vi "Configuration Utility.vi"() -> ()   [LabVIEW 2013, in "configuration library.lvlib"]
doc: "This is the main VI for the configuration editor."
uses:
  configuration library.lvlib
  Controls/StateCluster.ctl
  Configuration Editor/Classes/SystemConfigRepo/SystemConfigRepo.lvclass
  <vilib>/CEF_TreeControl/Node/NodeRef.ctl
  <vilib>/CEF_TreeControl/Node/NISE_CEF_Node.lvclass
  <vilib>/CEF_TreeControl/Node/UserEventRef.ctl
  <vilib>/CEF_TreeControl/Controls/EventCluster.ctl
  subVI/SplashScreen/splash screen.ctl
  subVI/SplashScreen/notifier data.ctl
  Controls/add message.ctl
  Controls/MoveMessage.ctl
  Configuration Editor/Classes/Systems/Systems.lvclass
  <vilib>/CEF_TreeControl/Repository/NISE_CEF_Repository.lvclass
  Configuration Editor/Classes/Module editor node/module editor node.lvclass
  <vilib>/NI/AMC/Create Single Message.vi
  <vilib>/NI/AMC/Update Message Routing Info.vi
  <vilib>/NI/AMC/Read Termination Message.vi
  Configuration Editor/subVIs/Glyphs Status.ctl
  Configuration Editor/subVIs/Add status to name.vi
  <vilib>/NI/AMC/Send Message.vi
  <vilib>/NI/AMC/Globals.vi
  Configuration Editor/Classes/EngineTags/EngineTags.lvclass
  Configuration Editor/Classes/Asynchronous Component Editor Node/Asynchronous Module Editor Node.lvclass
  <vilib>/NI/Module Timing Source/timing source/TBM timing source.lvclass
  Configuration Editor/Classes/TBM Configuration Node/TBM Configuration Node.lvclass
  <vilib>/NI/Tag Bus Module Framework/root configuration/TBM configuration.lvclass
  Framework Configuration Classes/target configuration/PL_Target Configuration.lvclass
  Configuration Editor/Classes/Targets/Targets.lvclass
  Configuration Editor/Classes/Engine Parent/Engine Parent Editor Node.lvclass
  Framework Configuration Classes/system configuration/PL_System Configuration.lvclass
  <vilib>/NI/Module Execution Interface/Engine Configuration/engine configuration.lvclass
  asynchronous execution module/configuration/asynchronous execution module configuration.lvclass
  <vilib>/NI/Tag Bus Module Framework/channel/TBM channel.lvclass
  <vilib>/NI/Tag Bus Module Framework/module configuration/TBM module configuration.lvclass
  <vilib>/NI/AMC/AMC.lvlib
  <vilib>/CEF_TreeControl/NISE_CEF_TreeControl.lvlib
  subVI/SplashScreen/splash screen.lvlib
  Framework Configuration Classes/class cache/PL_class cache.lvlib
panel:
  in  "Exit":bool
  in  "View":string(tree)
  # "Tag Bus Configuration Editor"
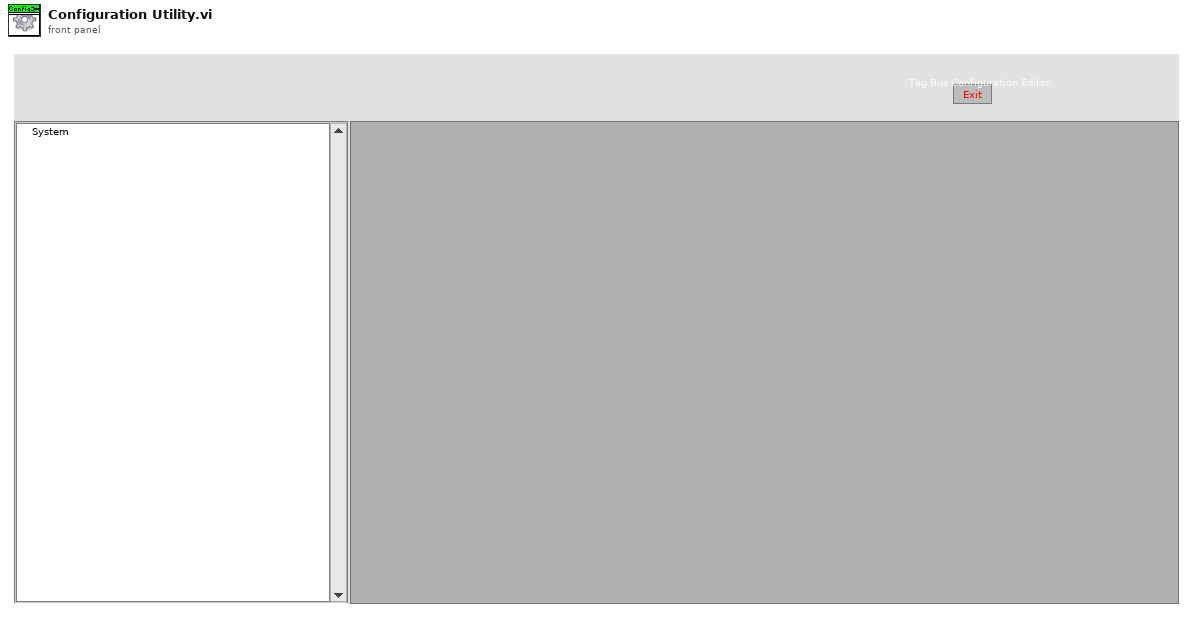
[diagram p1: front panel]
types:
  T1 = enum32{"Invalid", "Standard", "Closed", "Hidden", "Minimized", "Maximized"}
  T2 = typedef "configuration library.lvlib/StateCluster.ctl" = cluster{"repository":refnum<class "SystemConfigRepo.lvclass">, "root":T3, "unsaved changes":bool, "current path":path, "user event ref":T4, "glyph path":path[], "SplashScreen":T5, "classes cache":path}
  T3 = typedef "NISE_CEF_Node.lvclass/NodeRef.ctl" = refnum<data-value>
  T4 = typedef "NISE_CEF_Node.lvclass/UserEventRef.ctl" = refnum<user-event>
  T5 = typedef "configuration library.lvlib/splash screen.lvlib/splash screen.ctl" = cluster{"reference":refnum<vi>, "update notifier":refnum<notifier>, "Initialized":bool}
  T6 = typedef "AMC.lvlib/Message Queue.ctl" = refnum<queue>
  T7 = typedef "NISE_CEF_TreeControl.lvlib/EventCluster.ctl" = cluster{"command":string, "data":string}
  T8 = typedef "configuration library.lvlib/splash screen.lvlib/notifier data.ctl" = cluster{"Text":string, "percent":dbl}
  T9 = cluster{"node id":string, "RightClickPath":string}
  T10 = typedef "configuration library.lvlib/add message.ctl" = cluster{"node type":string, "to add to":string}
  T11 = typedef "configuration library.lvlib/MoveMessage.ctl" = cluster{"node ref":T3, "new parent":T3}
  T12 = typedef "configuration library.lvlib/FilePaths.ctl" = cluster{"glyphs":path[], "classes":path, "classes cache":path}
  T13 = typedef "PL_class cache.lvlib/cache definition.ctl" = cluster{"configuration":T14, "class cache data":T15}
  T14 = typedef "PL_class cache.lvlib/cache search configuration.ctl" = cluster{"Search Paths":path[], "Folders to Exclude":string[], "full class list":path[]}
  T15 = typedef "PL_class cache.lvlib/cached class information.ctl" = cluster{"targets":T16[], "engines":T17[], "modules":T17[], "ignored class list":path[]}
  T16 = typedef "PL_class cache.lvlib/target class metadata.ctl" = cluster{"file name":string, "fully qualified name":string, "menu display name":string, "configuration class name":string}
  T17 = typedef "PL_class cache.lvlib/class metadata.ctl" = cluster{"file name":string, "fully qualified name":string, "menu display name":string, "configuration class":string, "instances allowed":i32, "supported targets":T18[]}
  T18 = typedef "TBM configuration.lvclass/Target Types.ctl" = enum16{"Windows", "Mac", "Linux", "Linux RT ARM", "VxWorks", "Pharlap", "Other", "Linux RT x64"}
  T19 = typedef "NISE_CEF_Node.lvclass/Summary.ctl" = cluster{"ID":string, "parent ID":string, "node type":string, "text":string, "additional text":string, "glyph":string, "depth":i32}
  T20 = typedef "LVPoint32TypeDef.ctl" = cluster{"Horizontal":i32, "Vertical":i32}
  T21 = cluster{"data name":string, "drag data":variant}[]
  T22 = typedef "NISE_CEF_Node.lvclass/NodeMenuOptions.ctl" = cluster{"removable":bool, "movable":bool, "duplicate":bool}
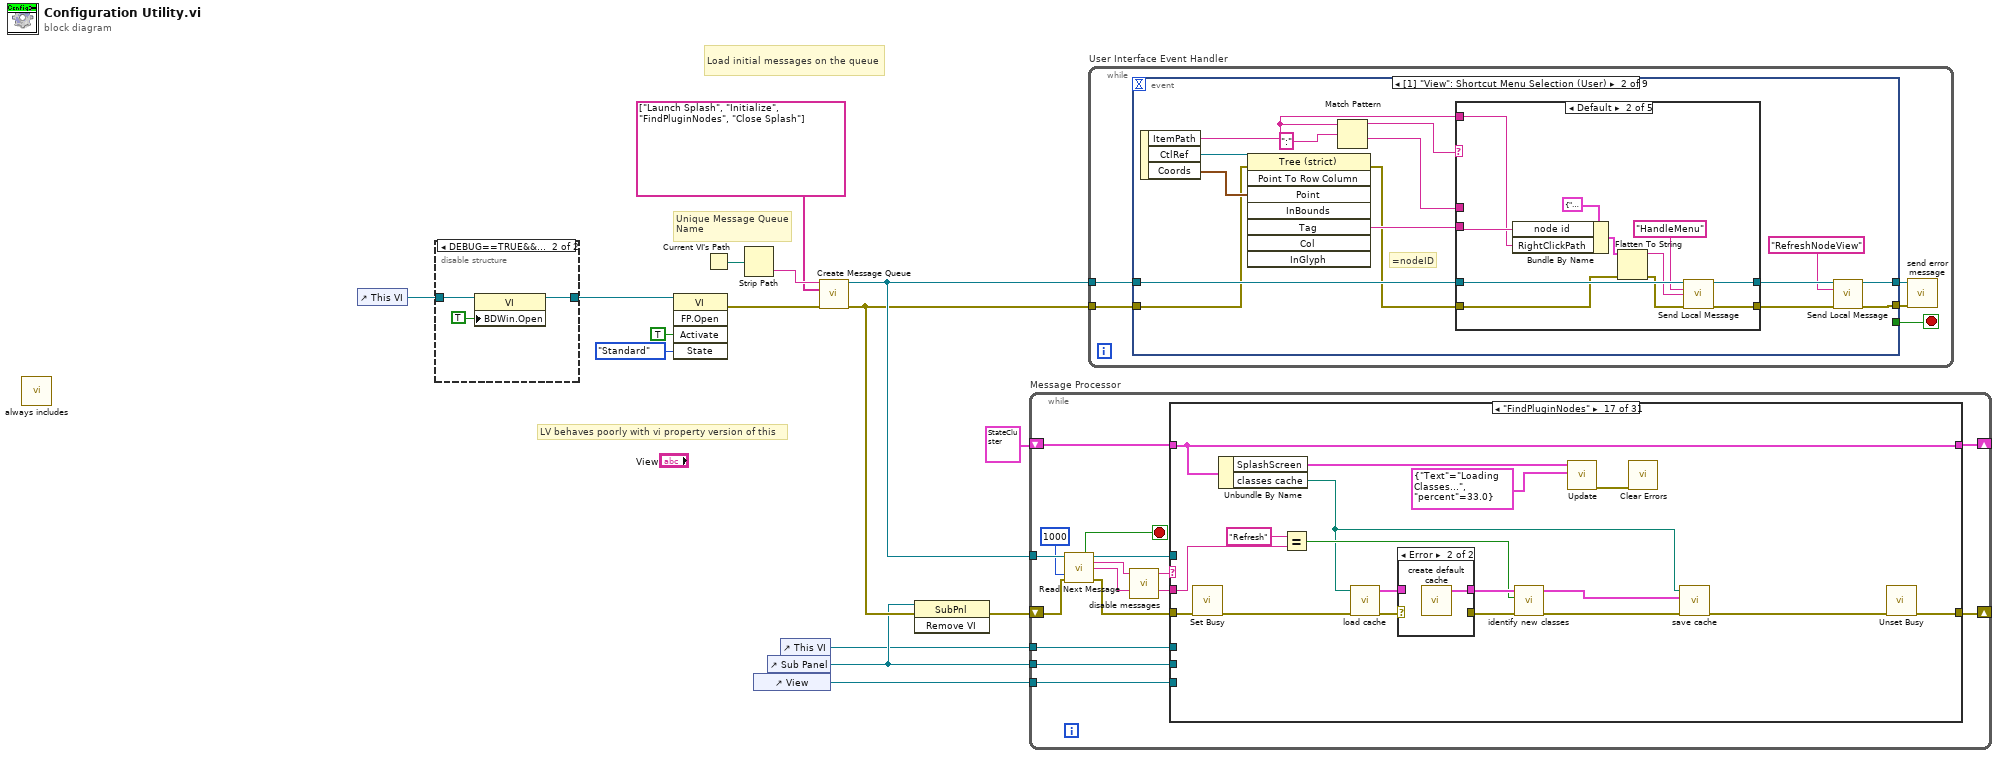
[diagram p0: block diagram]
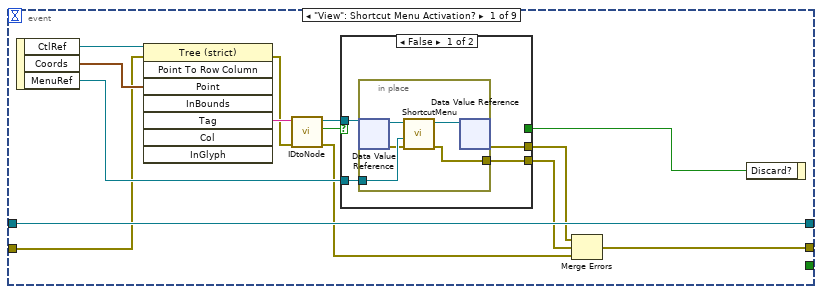
[diagram p3: hidden frame]
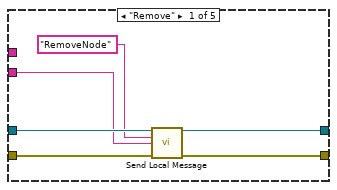
[diagram p5: hidden frame]
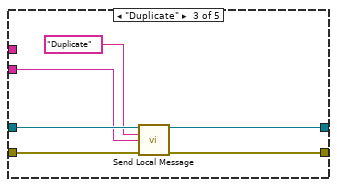
[diagram p6: hidden frame]
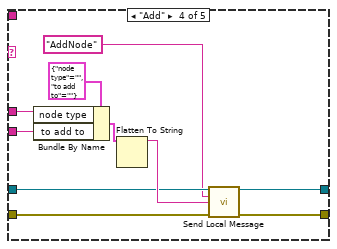
[diagram p7: hidden frame]
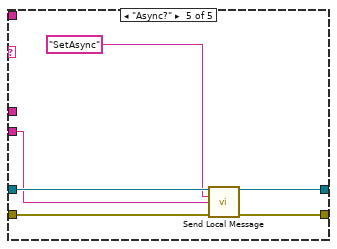
[diagram p8: hidden frame]
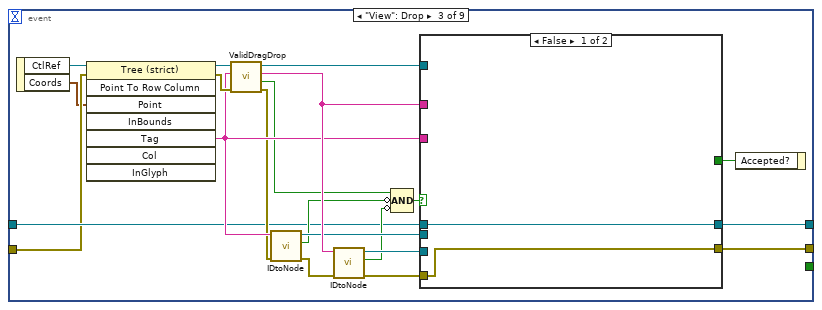
[diagram p9: hidden frame]
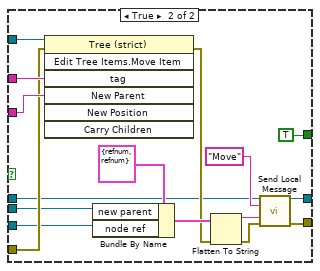
[diagram p10: hidden frame]
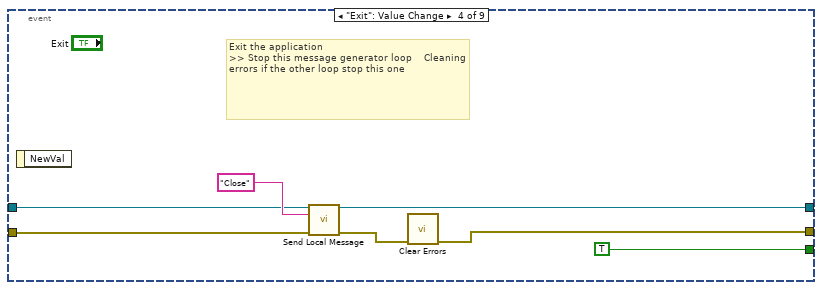
[diagram p11: hidden frame]
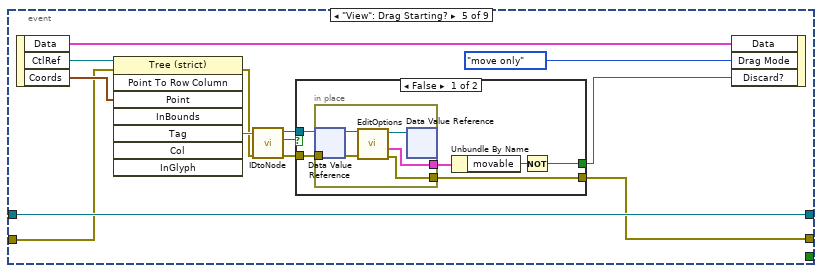
[diagram p12: hidden frame]
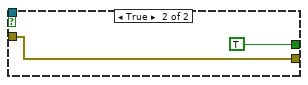
[diagram p13: hidden frame]
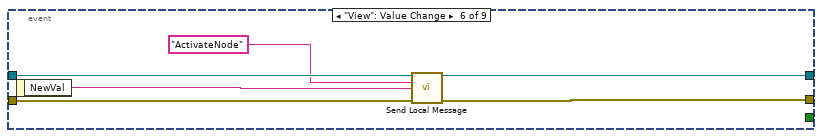
[diagram p14: hidden frame]
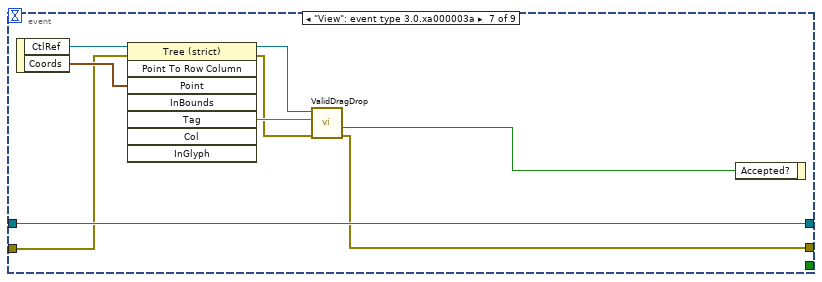
[diagram p15: hidden frame]
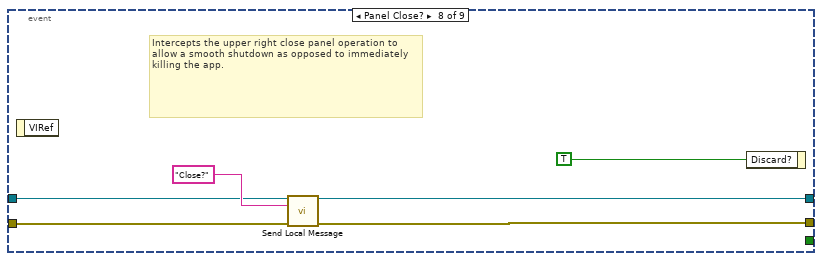
[diagram p16: hidden frame]
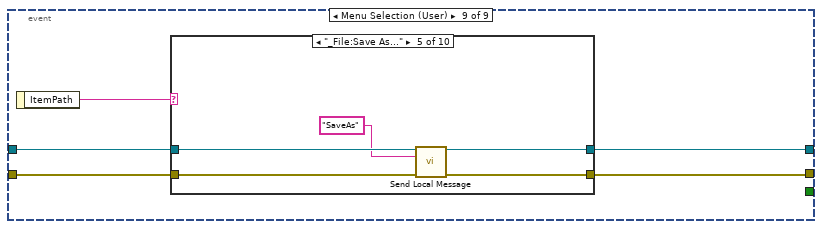
[diagram p17: hidden frame]
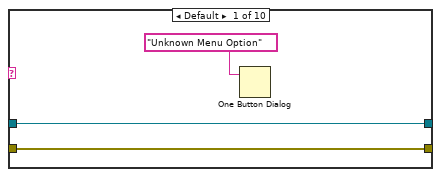
[diagram p18: hidden frame]
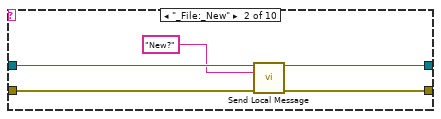
[diagram p19: hidden frame]
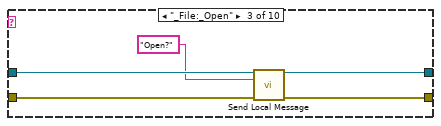
[diagram p20: hidden frame]
diagram:
  # "LV behaves poorly with vi property version of this"
  # "Unique Message Queue Name"
  # "Load initial messages on the queue"
  n1 = call "always includes.vi"() -> ()  [unwired: 12 in]
  n2 = control-ref of="This VI"() -> (w5:refnum<vi>)
  n3 = disable-structure shown="DEBUG==TRUE&&RUN_TIME_ENGINE==False" {
    disable-tunnel: [w16 w19] -> w6
    disable-tunnel: w5 -> [w16 w18]
    frame condition #0 {
    }
    frame condition #1 (active) {
      n4 = property class="VI"(reference=w18, "BDWin.Open"=TRUE ("Block Diagram Window:Open")) -> (reference out=w19:refnum<vi>)  [unwired: 1 in, 1 out]
    }
  }
  n5 = invoke class="VI" method="FP.Open"(reference=w6, "Activate"=TRUE ("Activate?"), "State"=T1."Standard") -> (error out=w9:errorcluster)  [unwired: 2 in, 4 out]
  n6 = Current VI's Path() -> (path=w14:path)
  n7 = Strip Path(path=w14) -> (name=w15:string)  [unwired: 1 out]
  n8 = control-ref of="View"() -> (w4:refnum<vi>)
  n9 = control-ref of="Sub Panel"() -> (w2:refnum<vi>)
  n10 = control-ref of="This VI"() -> (w1:refnum<vi>)
  n11 = call <vilib>:"Create Message Queue.vi"("message queue name"=w15, "initial message names"=string[] ["Launch Splash", "Initialize", "FindPluginNodes", "Close Splash"], "error in"=w9) -> ("message queue out"=w12:T6, "error out"=w10:errorcluster)  [unwired: 11 in]
  n12 = invoke class="SubPnl" method="Remove VI"(reference=w2, error in=w10) -> (error out=w3:errorcluster)  [unwired: 1 in, 2 out]
  n13 = while "Message Processor" {
    shift-right: [w32] -> _
    shift-left: w3 -> [w31]
    tunnel: w12 -> [w30]
    shift-right: [w28] -> _
    shift-left: T2 {"repository"=refnum, "root"=refnum, "unsaved changes"=FALSE, "current path"=path "", "user event ref"=refnum, "glyph path"=[], "SplashScreen"={"reference"=refnum, "update notifier"=refnum, "Initialized"=FALSE}, "classes cache"=path ""} -> [w27]
    tunnel: w1 -> [w22]
    tunnel: w2 -> [w21]
    tunnel: w4 -> [w20]
    stop <- w34 stop-if-true
    n14 = call <vilib>:"Read Next Message.vi"("message queue in"=w30, "timeout (1 ms)"=1000, "error in"=w31) -> ("exit process?"=w34:bool, "message queue out"=w26:T6, "message name"=w23:string, "message value"=w25:string, "error out"=w33:errorcluster)  [unwired: 5 in, 3 out]
    n15 = call "disable messages.vi"("message to check"=w23) -> ("message out"=w24:string)  [unwired: 10 in]
    n16 = case shown="\"FindPluginNodes\"" w24 {
      selector: w24 -> [_ w38 _ _ _ _ _ _ _ _ w138 _ _ w219 _ _ _ _ _ _ _ _ _ _ _ _ _ _ _ _ _]
      tunnel: w25 -> [_ _ _ _ _ _ _ w96 _ _ _ _ _ _ w239 _ w296 w304 w334 _ w372 w384 w402 _ w426 w461 _ _ w508 w531 _]
      tunnel: w33 -> [w36 w41 w43 w50 w67 w81 w87 w97 w123 w127 w135 w170 w182 w211 w244 w261 w294 w309 w336 w351 w370 w383 w403 w415 w427 w460 w486 w496 w507 w530 w536]
      tunnel: [w36 w41 w43 w53 w59 w82 w90 errorcluster {"status"=FALSE, "code"=0, "source"=""} ("error out") w121 w127 w140 w173 w175 w223 w243 w263 w281 w308 w327 w351 w371 w385 w406 w415 w430 w459 w482 w493 w506 w529 w535] -> w32
      tunnel: [w35 w37 w42 w51 w68 w72 w88 w98 w120 w126 w136 w171 w174 w224 w240 w262 w297 w305 w335 w350 w353 w386 w404 w416 w428 w453 w491 w495 w504 w532 w534] -> w28
      tunnel: w27 -> [w35 w37 w42 w52 w69 w73 w88 w98 w120 w126 w137 w169 w183 w218 w241 w262 w297 w306 w335 w350 w369 w386 w405 w417 w429 w453 w491 w495 w504 w532 w534]
      tunnel: w26 -> [_ _ _ _ _ w83 w89 w100 w122 _ w139 w172 w181 w222 w242 w264 _ w307 w323 _ _ _ _ _ _ _ _ _ w505 w528 _]
      tunnel: w22 -> [_ _ _ w44 w58 w70 _ _ _ _ _ _ _ _ _ _ _ _ _ _ _ _ _ _ _ _ w481 _ _ _ _]
      tunnel: w21 -> [_ _ _ _ _ _ _ w91 w113 _ _ _ _ w209 _ _ _ _ _ _ _ _ _ _ _ w454 _ w492 w497 _ _]
      tunnel: w20 -> [_ _ _ _ _ _ _ _ _ _ _ _ _ _ _ _ _ _ w322 _ w354 w379 w397 _ w425 w455 w485 _ _ _ _]
      frame "", "Idle" {
      }
      frame "Missing Message Handler", Default {
        # "Call this case if a message is received that is not handled by any other case. Typically this is a programming error as a result of a typo or unhandled message/missing message handler."
        n17 = Format Into String(format string="Internal Error: Missing message handler for '%s\" message." ("message"), w38) -> (resulting string=w40:string)  [unwired: 2 in, 1 out]
        n18 = One Button Dialog(message=w40) -> ()  [unwired: 2 out]
      }
      frame "------------Generic Operations------------" {
        # "Dummy case to add a seperation in the Case Structure menu"
      }
      frame "Launch Splash" {
        n19 = invoke class="VI" method="FP.Center"(reference=w44, error in=w50) -> (reference out=w48:refnum<vi>, error out=w47:errorcluster)  [unwired: 1 in, 1 out]
        n20 = invoke class="VI" method="FP.Open"(reference=w48, error in=w47, "State"=T1."Hidden") -> (error out=w45:errorcluster)  [unwired: 2 in, 4 out]
        n21 = call "Launch.vi"("error in"=w45) -> ("error out"=w53:errorcluster, "SplashScreen"=w49:T5)  [unwired: 9 in]
        n22 = Bundle By Name(cluster=w52, "SplashScreen"=w49) -> (w51:T2)
      }
      frame "Initialize" {
        # "issues in exe"
        n23 = Current VI's Menubar() -> (w66:refnum<k9>)
        n24 = call "menu options.vi"("error in"=w67, "VI ref"=w58, "menu ref in"=w66) -> ("error out"=w63:errorcluster)  [unwired: 7 in, 1 out]
        n25 = Create User Event(user event datatype=T7 {"command"="", "data"=""} ("Event"), error in=w63) -> (user event=w64:refnum<user-event>, error out=w57:errorcluster)
        n26 = call "default file paths.vi"() -> ("paths"=w65:T12)  [unwired: 11 in]
        n27 = Unbundle By Name(w65) -> ("classes cache"=w56:path, "glyphs"=w60:path[])
        n28 = Type Cast(type=T4 refnum ("user event ref"), x=w64) -> (*(type *) &x=w55:T4)
        n29 = control-ref of="View"() -> (w61:refnum<vi>)
        n30 = Bundle By Name(cluster=w69, "user event ref"=w55, "classes cache"=w56, "glyph path"=w60) -> (w68:T2)
        n31 = call "Load Custom Status Glyph.vi"("tree ref"=w61, "error in"=w57, "glyph directories"=w60) -> ("error out"=w59:errorcluster)  [unwired: 8 in]
      }
      frame "Close Splash" {
        n32 = Unbundle By Name(w73) -> ("SplashScreen"=w79:T5)
        n33 = call "Close.vi"("error in"=w81, "SplashScreen"=w79) -> ("error out"=w75:errorcluster, "SplashScreen out"=w71:T5)  [unwired: 8 in]
        n34 = Bundle By Name(cluster=w73, "SplashScreen"=w71) -> (w72:T2)
        n35 = invoke class="VI" method="FP.Open"(reference=w70, error in=w75, "State"=T1."Standard") -> (reference out=w77:refnum<vi>, error out=w76:errorcluster)  [unwired: 2 in, 3 out]
        n36 = Close Reference(reference=w77, error in (no error)=w76) -> (error out=w74:errorcluster)
        n37 = call <vilib>:"Send Local Message.vi"("message queue in"=w83, "message name"="New" ("Message Name"), "error in"=w74) -> ("error out"=w82:errorcluster)  [unwired: 10 in, 2 out]
      }
      frame "Close" {
        n38 = Unbundle By Name(w88) -> ("root"=w85:T3)
        n39 = call <vilib>:"CloseNode.vi"("error in"=w87, "node ref"=w85) -> ("error out"=w84:errorcluster)  [unwired: 9 in]
        n40 = call <vilib>:"Send Local Message.vi"("message queue in"=w89, "message name"="Exit", "error in"=w84) -> ("error out"=w90:errorcluster)  [unwired: 10 in, 2 out]
      }
      frame "Error" {
        n41 = Unbundle By Name(w98) -> ("user event ref"=w94:T4)
        n42 = call "Remove UI without races.vi"("error in"=w97, "user event ref"=w94, "sub panel ref in"=w91) -> ("error out"=w92:errorcluster)  [unwired: 7 in, 1 out]
        n43 = case shown="\"\"" w96 {
          selector: w96 -> [w102 _]
          tunnel: w97 -> [w103 w104]
          tunnel: [w101 w104] -> w93
          frame Default {
            n44 = Unflatten From String(type=w103, binary string=w102, error in (no error)=w103) -> (value=w101:errorcluster)  [unwired: 2 in, 2 out]
          }
          frame "" {
          }
        }
        n45 = call <vilib>:"Clear Errors.vi"("error in (no error)"=w92) -> ()  [unwired: 6 in, 1 out]
        n46 = Unbundle By Name(w93) -> ("code"=w95:i32)
        n47 = case shown="15550" w95 {
          tunnel: w100 -> [_ _ _ w110 _]
          tunnel: w93 -> [_ _ _ w109 w112]
          frame -2147220623, -2147220621, -2147220364, 56, 63 {
            n48 = One Button Dialog(message="Problem communicating with remote device.  Make sure a valid device is selected and that the IP address is correct.") -> ()  [unwired: 1 in, 1 out]
          }
          frame 1003 {
            n49 = One Button Dialog(message="Dev Error: The Ui.vi for the selected class is broken") -> ()  [unwired: 1 in, 1 out]
          }
          frame 15550 {
            n50 = One Button Dialog(message="The cRIO does not yet have a configuration to download. Create or open a configuration and download it to the cRIO") -> ()  [unwired: 1 in, 1 out]
          }
          frame 537549 {
            n51 = call <vilib>:"Send Local Message.vi"("message queue in"=w110, "message name"="Exit", "error in"=w109) -> ()  [unwired: 10 in, 3 out]
            n52 = One Button Dialog(message="Invalid configuration file.") -> ()  [unwired: 1 in, 1 out]
          }
          frame 1, Default {
            n53 = call <vilib>:"Simple Error Handler.vi"("error in (no error)"=w112) -> ()  [unwired: 1 in, 8 out]
          }
        }
      }
      frame "Exit" {
        # "Stop the VI                                                                             >> Perform any cleanup tasks in this message case. >> Clear display before closing."
        n54 = call <vilib>:"Destroy Message Queue.vi"("message queue in"=w122, "error in"=w123) -> ("error out"=w117:errorcluster)  [unwired: 11 in, 2 out]
        n55 = control-ref of="Exit"() -> (w119:refnum<vi>)
        n56 = Unbundle By Name(w120) -> ("user event ref"=w114:T4)
        n57 = property class="Bool (strict)"(reference=w119, error in=w117, "Val(Sgnl)"=FALSE ("Exit")) -> (error out=w116:errorcluster)  [unwired: 1 out]
        n58 = call "Remove UI without races.vi"("error in"=w116, "user event ref"=w114, "sub panel ref in"=w113) -> ("error out"=w115:errorcluster)  [unwired: 7 in, 1 out]
        n59 = disable-structure shown="RUN_TIME_ENGINE==True" {
          disable-tunnel: [w124 w125] -> w121
          disable-tunnel: w115 -> [w124 w125]
          frame condition #0 (active) {
          }
          frame condition #1 {
            n60 = Quit LabVIEW() -> ()  [unwired: 1 in]
          }
        }
      }
      frame "------------Menu Operations--------------" {
        # "Dummy case to add a seperation in the Case Structure menu"
      }
      frame "Close?", "New?", "Open?" {
        n61 = Unbundle By Name(w137) -> ("unsaved changes"=w128:bool, "user event ref"=w129:T4)
        n62 = case shown="False" w128 {
          tunnel: [TRUE ("SaveFlag") w156] -> w131
          tunnel: w137 -> [w150 w155]
          tunnel: [w150 w154] -> w136
          tunnel: w135 -> [w149 w153]
          tunnel: [w149 w152] -> w130
          frame False {
            # "If there is nothing to save Go do Action"
          }
          frame True {
            n63 = call "dialog save dirty dot.vi"("error in"=w153, "state in"=w155) -> ("error out"=w152:errorcluster, "new"=w156:bool, "state out"=w154:T2)  [unwired: 7 in]
          }
        }
        n64 = Search and Replace String(input string=w138, search string="?", replace string="") -> (result string=w132:string)  [unwired: 5 in, 3 out]
        n65 = case shown="True" w131 {
          tunnel: w130 -> [w141 w148]
          tunnel: [w141 w144] -> w140
          tunnel: w139 -> [_ w147]
          tunnel: w132 -> [_ w146]
          tunnel: w129 -> [_ w143]
          frame False {
          }
          frame True {
            n66 = control-ref of="Sub Panel"() -> (w142:refnum<vi>)
            n67 = call <vilib>:"Send Local Message.vi"("message queue in"=w147, "message name"=w146, "error in"=w148) -> ("error out"=w145:errorcluster)  [unwired: 10 in, 2 out]
            n68 = call "Remove UI without races.vi"("error in"=w145, "user event ref"=w143, "sub panel ref in"=w142) -> ("error out"=w144:errorcluster)  [unwired: 7 in, 1 out]
          }
        }
      }
      frame "New" {
        # "unused"
        n69 = call "create default cache.vi"() -> ("cache"=w159:T13)  [unwired: 11 in]
        n70 = Unbundle By Name(w159) -> ("configuration.Search Paths"=w158:path[])
        n71 = call-dynamic "Initialize.vi"("error in"=w170, "node in"=refnum<class "Systems.lvclass"> refnum ("Systems.lvclass")) -> ("error out"=w165:errorcluster, "data value reference"=w166:T3)  [unwired: 7 in, 1 out]
        n72 = Delete From Array(array=w158) -> (deleted portion=w157:path)  [unwired: 2 in, 1 out]
        n73 = call-dynamic "Initialize.vi"("error in"=w165, "path"=w157, "repository in"=refnum<class "SystemConfigRepo.lvclass"> refnum ("SystemConfigRepo.lvclass")) -> ("error out"=w164:errorcluster, "repository out"=w163:refnum<class "SystemConfigRepo.lvclass">)  [unwired: 7 in]
        n74 = Bundle By Name(cluster=w169, "unsaved changes"=FALSE ("SaveFlag"), "repository"=w163, "root"=w166, "current path"=path "") -> (w171:T2)
        n75 = call <vilib>:"Send Local Message.vi"("message queue in"=w172, "message name"="PopulateTree", "error in"=w164) -> ("error out"=w173:errorcluster)  [unwired: 10 in, 2 out]
      }
      frame "Open" {
        n76 = call <vilib>:"Set Busy.vi"() -> ("error out"=w178:errorcluster)  [unwired: 10 in, 1 out]
        n77 = call "File Dialog"("pattern (all files)"="*.pcfg") -> ("selected path"=w180:path, "cancelled"=w179:bool)  [unwired: 11 in, 2 out]
        n78 = case shown="False" w179 {
          tunnel: w183 -> [w192 w208]
          tunnel: [w191 w208] -> w174
          tunnel: w182 -> [w190 w207]
          tunnel: w181 -> [w189 _]
          tunnel: [w188 w207] -> w175
          tunnel: w180 -> [w185 _]
          tunnel: w178 -> [w184 w206]
          tunnel: [w184 w206] -> w177
          frame False {
            n79 = in-place {
              in-place-border: w190 -> [w205]
              in-place-border: [w194] -> w186
              in-place-border: w185 -> [w200]
              n80 = in-place-cluster #1(w192) -> ("repository"=w193:refnum<class "SystemConfigRepo.lvclass">, "current path"=w201:path)  [unwired: 2 out]
              n81 = call-dynamic "Open.vi"("error in"=w205, "file path"=w200, "SystemConfigRepo in"=w193) -> ("error out"=w202:errorcluster, "SystemConfigRepo out"=w198:refnum<class "SystemConfigRepo.lvclass">)  [unwired: 6 in, 1 out]
              n82 = call-dynamic "WriteTree.vi"("error in"=w202, "SystemConfigRepo in"=w198) -> ("error out"=w195:errorcluster, "root"=w203:T3, "repository out"=w197:refnum<class "NISE_CEF_Repository.lvclass">)  [unwired: 7 in]
              n83 = To More Specific Class(target class=w193, reference=w197, error in=w195) -> (specific class reference=w196:refnum<class "SystemConfigRepo.lvclass">, error out=w194:errorcluster)
              n84 = Select(t=w201, s=w194, f=w200) -> (s? t:f=w199:path)
              n85 = in-place-cluster #1("unsaved changes"=FALSE ("SaveFlag"), "repository"=w196, "root"=w203, "current path"=w199) -> (w191:T2)
            }
            n86 = call <vilib>:"Send Local Message.vi"("message queue in"=w189, "message name"="PopulateTree", "error in"=w186) -> ("error out"=w188:errorcluster)  [unwired: 10 in, 2 out]
          }
          frame True {
          }
        }
        n87 = call <vilib>:"Unset Busy.vi"("error in (no error)"=w177) -> ()  [unwired: 10 in, 1 out]
      }
      frame "Save", "SaveAs" {
        n88 = Unbundle By Name(w218) -> ("user event ref"=w212:T4)
        n89 = call <vilib>:"Set Busy.vi"() -> ("error out"=w216:errorcluster)  [unwired: 10 in, 1 out]
        n90 = call "Remove UI without races.vi"("error in"=w211, "user event ref"=w212, "sub panel ref in"=w209) -> ("error out"=w210:errorcluster)  [unwired: 7 in, 1 out]
        n91 = flat-sequence {
          tunnel: w210 -> [w231]
          tunnel: w219 -> [w229]
          tunnel: w218 -> [w226]
          tunnel: w216 -> [w225]
          tunnel: [w232] -> w215
          tunnel: [w230] -> w214
          tunnel: [w225] -> w213
          tunnel: [w234] -> w217
          tunnel: [w235] -> w220
          tunnel: [w236] -> w224
          tunnel: w215 -> [w236]
          tunnel: w214 -> [w235]
          tunnel: w213 -> [w234]
          frame #0 {
            n92 = Equal?(x="SaveAs", y=w229) -> (x = y?=w228:bool)
            n93 = call "save operation.vi"("force save as"=w228, "error in"=w231, "state cluster"=w226) -> ("error out"=w230:errorcluster, "state out"=w232:T2)  [unwired: 7 in]
          }
          frame #1 {
            n94 = local read "View"() -> (w233:string)
            n95 = property on="View" class="Tree (strict)"("Val(Sgnl)"=w233) -> ()  [unwired: 2 in, 2 out]
          }
        }
        n96 = call <vilib>:"Unset Busy.vi"("error in (no error)"=w217) -> ()  [unwired: 10 in, 1 out]
        n97 = call <vilib>:"Send Local Message.vi"("message queue in"=w222, "message name"="PopulateTree", "error in"=w220) -> ("error out"=w223:errorcluster)  [unwired: 10 in, 2 out]
      }
      frame "Custom View" {
        n98 = in-place {
          in-place-border: w244 -> [w257]
          in-place-border: [w248] -> w237
          in-place-border: w239 -> [w249]
          n99 = in-place-cluster #2(w241) -> ("repository"=w246:refnum<class "SystemConfigRepo.lvclass">, "root"=w255:T3)
          n100 = call-dynamic "ReadTree.vi"("error in"=w257, "root"=w255, "SystemConfigRepo in"=w246) -> ("error out"=w253:errorcluster, "repository out"=w251:refnum<class "NISE_CEF_Repository.lvclass">)  [unwired: 7 in]
          n101 = call-dynamic "CustomView.vi"("error in"=w253, "view name"=w249, "repository in"=w251) -> ("error out"=w252:errorcluster, "repository out"=w250:refnum<class "NISE_CEF_Repository.lvclass">)  [unwired: 7 in]
          n102 = call-dynamic "WriteTree.vi"("error in"=w252, "repository in"=w250) -> ("error out"=w256:errorcluster, "root"=w254:T3, "repository out"=w247:refnum<class "NISE_CEF_Repository.lvclass">)  [unwired: 7 in]
          n103 = To More Specific Class(target class=w246, reference=w247, error in=w256) -> (specific class reference=w245:refnum<class "SystemConfigRepo.lvclass">, error out=w248:errorcluster)
          n104 = in-place-cluster #2("repository"=w245, "root"=w254) -> (w240:T2)
        }
        n105 = call <vilib>:"Send Local Message.vi"("message queue in"=w242, "message name"="PopulateTree", "error in"=w237) -> ("error out"=w243:errorcluster)  [unwired: 10 in, 2 out]
      }
      frame "Edit Plugin Search Paths" {
        n106 = Unbundle By Name(w262) -> ("classes cache"=w258:path)
        n107 = call "load cache.vi"("error in"=w261, "cache path"=w258) -> ("error out"=w259:errorcluster, "cache"=w260:T13)  [unwired: 8 in]
        n108 = Unbundle By Name(w260) -> ("configuration.Search Paths"=w268:path[])
        n109 = call "dialog edit search paths.vi"("error in"=w259, "Plugin Search Paths"=w268) -> ("error out"=w265:errorcluster, "Cancelled?"=w267:bool, "Plugin Search Paths"=w266:path[])  [unwired: 7 in]
        n110 = case shown="False" w267 {
          tunnel: w260 -> [w278 _]
          tunnel: w266 -> [w277 _]
          tunnel: w265 -> [w271 w279]
          tunnel: w264 -> [w274 _]
          tunnel: [w273 w279] -> w263
          tunnel: w258 -> [w269 _]
          frame False {
            n111 = Bundle By Name(cluster=w278, "configuration.Search Paths"=w277) -> (w270:T13)
            n112 = call "save cache.vi"("error in"=w271, "cache"=w270, "path"=w269) -> ("error out"=w272:errorcluster)  [unwired: 8 in]
            n113 = call <vilib>:"Send Local Message.vi"("message queue in"=w274, "message name"="FindPluginNodes", "message value"="Refresh", "error in"=w272) -> ("error out"=w273:errorcluster)  [unwired: 9 in, 2 out]
          }
          frame True {
          }
        }
      }
      frame "FindPluginNodes" {
        n114 = call <vilib>:"Set Busy.vi"("error in (no error)"=w294) -> ("error out"=w293:errorcluster)  [unwired: 9 in, 1 out]
        n115 = Unbundle By Name(w297) -> ("SplashScreen"=w287:T5, "classes cache"=w283:path)
        n116 = Equal?(x="Refresh", y=w296) -> (x = y?=w288:bool)
        n117 = call "load cache.vi"("error in"=w293, "cache path"=w283) -> ("error out"=w292:errorcluster, "cache"=w291:T13)  [unwired: 8 in]
        n118 = case shown="Error" w292 {
          selector: w292 -> [w300 _]
          tunnel: [w298 w301] -> w289
          tunnel: w291 -> [w299 _]
          tunnel: [w300 _] -> w290
          frame No Error {
            n119 = call "remove missing files.vi"("cache in"=w299) -> ("cache out"=w298:T13)  [unwired: 10 in]
          }
          frame Error {
            n120 = call "create default cache.vi"() -> ("cache"=w301:T13)  [unwired: 11 in]
          }
        }
        n121 = call "identify new classes.vi"("error in"=w290, "force scan"=w288, "cache in"=w289) -> ("error out"=w284:errorcluster, "cache out"=w280:T13)  [unwired: 7 in]
        n122 = call "Update.vi"("Update"=T8 {"Text"="Loading Classes...", "percent"=33.0}, "SplashScreen in"=w287) -> ("error out"=w286:errorcluster)  [unwired: 8 in, 1 out]
        n123 = call <vilib>:"Clear Errors.vi"("error in (no error)"=w286) -> ()  [unwired: 6 in, 1 out]
        n124 = call "save cache.vi"("error in"=w284, "cache"=w280, "path"=w283) -> ("error out"=w282:errorcluster)  [unwired: 8 in]
        n125 = call <vilib>:"Unset Busy.vi"("error in (no error)"=w282) -> ("error out"=w281:errorcluster)  [unwired: 10 in]
      }
      frame "Test" {
        n126 = in-place {
          in-place-border: w309 -> [w321]
          in-place-border: [w316] -> w302
          in-place-border: w304 -> [_]
          n127 = in-place-cluster #3(w306) -> ("repository"=w311:refnum<class "SystemConfigRepo.lvclass">, "root"=w318:T3)
          n128 = call-dynamic "ReadTree.vi"("error in"=w321, "root"=w318, "SystemConfigRepo in"=w311) -> ("error out"=w317:errorcluster, "repository out"=w313:refnum<class "NISE_CEF_Repository.lvclass">)  [unwired: 7 in]
          n129 = To More Specific Class(target class=w311, reference=w313, error in=w317) -> (specific class reference=w312:refnum<class "SystemConfigRepo.lvclass">, error out=w314:errorcluster)
          n130 = call-dynamic "WriteTree.vi"("error in"=w314, "SystemConfigRepo in"=w312) -> ("error out"=w320:errorcluster, "root"=w319:T3, "repository out"=w315:refnum<class "NISE_CEF_Repository.lvclass">)  [unwired: 7 in]
          n131 = To More Specific Class(target class=w311, reference=w315, error in=w320) -> (specific class reference=w310:refnum<class "SystemConfigRepo.lvclass">, error out=w316:errorcluster)
          n132 = in-place-cluster #3("repository"=w310, "root"=w319) -> (w305:T2)
        }
        n133 = call <vilib>:"Send Local Message.vi"("message queue in"=w307, "message name"="PopulateTree", "error in"=w302) -> ("error out"=w308:errorcluster)  [unwired: 10 in, 2 out]
      }
      frame "HandleMenu" {
        n134 = Unflatten From String(type=T9 {"node id"="", "RightClickPath"=""} ("input cluster"), binary string=w334, error in (no error)=w336) -> (value=w332:T9, error out=w331:errorcluster)  [unwired: 2 in, 1 out]
        n135 = Unbundle By Name(w332) -> ("RightClickPath"=w325:string, "node id"=w330:string)
        n136 = call <vilib>:"IDtoNode.vi"("error in"=w331, "ID"=w330) -> ("error out"=w328:errorcluster, "node ref"=w329:T3)  [unwired: 7 in, 1 out]
        n137 = in-place {
          in-place-border: w328 -> [w349]
          in-place-border: [w344] -> w327
          in-place-border: [w343] -> w326
          in-place-border: w325 -> [w342]
          in-place-border: [w342] -> w324
          in-place-border: w323 -> [w341]
          in-place-border: w322 -> [w340]
          n138 = in-place-dvr #4(w329) -> (w346:refnum<class "NISE_CEF_Node.lvclass">, w348:errorcluster)
          n139 = Merge Errors(w349, w348) -> (w347:errorcluster)
          n140 = call-dynamic "MenuHandler.vi"("tree control"=w340, "message queue out"=w341, "error in (no error)"=w347, "menu string"=w342, "NISE_CEF_Node in"=w346) -> ("error out"=w344:errorcluster, "Unhandled"=w343:bool, "NISE_CEF_Node out"=w345:refnum<class "NISE_CEF_Node.lvclass">)  [unwired: 4 in]
          n141 = in-place-dvr #4(w345) -> ()  [unwired: 2 out]
        }
        n142 = case shown="True" w326 {
          tunnel: w324 -> [_ w337]
          frame False {
          }
          frame True {
            n143 = Concatenate Strings("Unknown item path:\n" ("message"), w337) -> (w339:string)
            n144 = One Button Dialog(message=w339) -> ()  [unwired: 1 in, 1 out]
          }
        }
      }
      frame "-------TreeControl Operations-----------" {
        # "Dummy case to add a seperation in the Case Structure menu"
      }
      frame "AddNode" {
        n145 = call <vilib>:"Set Busy.vi"("error in (no error)"=w370) -> ("error out"=w355:errorcluster)  [unwired: 9 in, 1 out]
        n146 = Unflatten From String(type=T10 {"node type"="", "to add to"=""} ("input cluster"), binary string=w372) -> (value=w365:T10)  [unwired: 3 in, 2 out]
        n147 = Unbundle By Name(w365) -> ("to add to"=w362:string, "node type"=w358:string)
        n148 = in-place {
          in-place-border: w358 -> [w378]
          in-place-border: [w375] -> w357
          in-place-border: w355 -> [w374]
          in-place-border: [w373] -> w356
          n149 = in-place-cluster #5(w369) -> ("repository"=w377:refnum<class "SystemConfigRepo.lvclass">)
          n150 = call-dynamic "GetClassPath.vi"("error in"=w374, "class name"=w378, "SystemConfigRepo in"=w377) -> ("error out"=w373:errorcluster, "class path"=w375:path, "SystemConfigRepo out"=w376:refnum<class "SystemConfigRepo.lvclass">)  [unwired: 6 in]
          n151 = in-place-cluster #5("repository"=w376) -> (w353:T2)
        }
        n152 = call <vilib>:"Get LV Class Default Value.vi"("error in (no error)"=w356, "class path"=w357) -> ("error out"=w367:errorcluster, "object"=w368:refnum<class>)  [unwired: 8 in]
        n153 = To More Specific Class(target class=refnum<class "NISE_CEF_Node.lvclass"> refnum ("NISE_CEF_Node.lvclass"), reference=w368, error in=w367) -> (specific class reference=w364:refnum<class "NISE_CEF_Node.lvclass">, error out=w361:errorcluster)
        n154 = call <vilib>:"AddNode.vi"("error in"=w361, "node in"=w364, "parent node ID"=w362) -> ("error out"=w360:errorcluster, "summary"=w359:T19[])  [unwired: 7 in]
        n155 = call <vilib>:"PopulateTreeSumary.vi"("error in"=w360, "array"=w359, "tree ref in"=w354) -> ("error out"=w352:errorcluster)  [unwired: 8 in]
        n156 = call <vilib>:"Unset Busy.vi"("error in (no error)"=w352) -> ("error out"=w371:errorcluster)  [unwired: 10 in]
      }
      frame "Duplicate" {
        n157 = call <vilib>:"IDtoNode.vi"("error in"=w383, "ID"=w384) -> ("error out"=w381:errorcluster, "invalid Id"=w380:bool, "node ref"=w382:T3)  [unwired: 7 in]
        n158 = case shown="False" w380 {
          tunnel: [w395 w396] -> w385
          tunnel: w382 -> [w394 _]
          tunnel: w381 -> [w391 w396]
          tunnel: w379 -> [w387 _]
          frame False {
            n159 = call <vilib>:"DuplicateNode.vi"("same parent?"=TRUE ("s"), "error in"=w391, "node ref in"=w394) -> ("error out"=w392:errorcluster, "new node ref"=w393:T3)  [unwired: 7 in]
            n160 = call <vilib>:"Summary.vi"("error in"=w392, "node self ref"=w393) -> ("error out"=w389:errorcluster, "summary"=w388:T19[])  [unwired: 8 in]
            n161 = call <vilib>:"PopulateTreeSumary.vi"("error in"=w389, "array"=w388, "tree ref in"=w387) -> ("error out"=w395:errorcluster)  [unwired: 8 in]
          }
          frame True {
          }
        }
      }
      frame "RefreshNode" {
        # "Refreshes the node in the Tree               Sets the save flag to true                       This case can be called from the UIs of the nodes"
        n162 = call <vilib>:"IDtoNode.vi"("error in"=w403, "ID"=w402) -> ("error out"=w400:errorcluster, "invalid Id"=w398:bool, "node ref"=w399:T3)  [unwired: 7 in]
        n163 = case shown="False" w398 {
          tunnel: [w412 w413] -> w406
          tunnel: w400 -> [w409 w413]
          tunnel: w399 -> [w408 _]
          tunnel: w397 -> [w407 _]
          frame False {
            n164 = call <vilib>:"Summary.vi"("error in"=w409, "node self ref"=w408) -> ("error out"=w411:errorcluster, "summary"=w410:T19[])  [unwired: 8 in]
            n165 = call <vilib>:"RefreshSubTree.vi"("error in"=w411, "node information"=w410, "tree ref in"=w407) -> ("error out"=w412:errorcluster)  [unwired: 7 in, 1 out]
          }
          frame True {
          }
        }
        n166 = Bundle By Name(cluster=w405, "unsaved changes"=TRUE ("SaveFlag")) -> (w404:T2)
      }
      frame "SetDirtyDot" {
        n167 = Bundle By Name(cluster=w417, "unsaved changes"=TRUE ("SaveFlag")) -> (w416:T2)
      }
      frame "SetAsync" {
        # "Refreshes the node in the Tree               Sets the save flag to true                       This case can be called from the UIs of the nodes"
        n168 = call <vilib>:"IDtoNode.vi"("error in"=w427, "ID"=w426) -> ("error out"=w421:errorcluster, "invalid Id"=w423:bool, "node ref"=w422:T3)  [unwired: 7 in]
        n169 = To More Specific Class(target class=refnum<data-value> refnum, reference=w422, error in=w421) -> (specific class reference=w419:refnum<data-value>, error out=w418:errorcluster)
        n170 = case shown="False" w423 {
          tunnel: [w437 w451] -> w430
          tunnel: w418 -> [w432 w451]
          tunnel: w419 -> [w436 _]
          tunnel: w425 -> [w438 _]
          frame False {
            n171 = in-place {
              in-place-border: w432 -> [w450]
              in-place-border: [w443] -> w431
              n172 = in-place-dvr #6(w436) -> (w446:refnum<class "module editor node.lvclass">, w449:errorcluster)
              n173 = Merge Errors(w450, w449) -> (w445:errorcluster)
              n174 = call-dynamic "Read Asynchronous_.vi"("error in"=w445, "Module Editor Node in"=w446) -> ("error out"=w444:errorcluster, "Asynchronous?"=w442:bool, "Module Editor Node out"=w447:refnum<class "module editor node.lvclass">)  [unwired: 7 in]
              n175 = Not(x=w442) -> (.not. x?=w441:bool)
              n176 = call-dynamic "Write Asynchronous_.vi"("error in"=w444, "Asynchronous?"=w441, "Module Editor Node in"=w447) -> ("error out"=w443:errorcluster, "Module Editor Node out"=w448:refnum<class "module editor node.lvclass">)  [unwired: 7 in]
              n177 = in-place-dvr #6(w448) -> (w435:refnum<data-value>, w434:errorcluster)
            }
            n178 = Merge Errors(w431, w434) -> (w433:errorcluster)
            n179 = call <vilib>:"Summary.vi"("error in"=w433, "node self ref"=w435) -> ("error out"=w440:errorcluster, "summary"=w439:T19[])  [unwired: 8 in]
            n180 = call <vilib>:"RefreshSubTree.vi"("error in"=w440, "node information"=w439, "tree ref in"=w438) -> ("error out"=w437:errorcluster)  [unwired: 7 in, 1 out]
          }
          frame True {
          }
        }
        n181 = Bundle By Name(cluster=w429, "unsaved changes"=TRUE ("SaveFlag")) -> (w428:T2)
      }
      frame "RemoveNode" {
        n182 = Unbundle By Name(w453) -> ("user event ref"=w452:T4)
        n183 = call <vilib>:"IDtoNode.vi"("error in"=w460, "ID"=w461) -> ("error out"=w458:errorcluster, "invalid Id"=w456:bool, "node ref"=w457:T3)  [unwired: 7 in]
        n184 = case shown="True" w456 {
          tunnel: w458 -> [w469 w479]
          tunnel: w457 -> [w467 _]
          tunnel: [w471 w479] -> w459
          tunnel: w455 -> [w470 _]
          tunnel: w454 -> [w466 _]
          tunnel: w452 -> [w465 _]
          frame False {
            n185 = call "check if subpanel should be closed.vi"("error in"=w469, "SubPanel in"=w466, "node in"=w467) -> ("error out"=w464:errorcluster, "needs closing"=w462:bool, "node out"=w468:T3)  [unwired: 6 in]
            n186 = case shown="True" w462 {
              tunnel: w466 -> [_ w478]
              tunnel: w465 -> [_ w477]
              tunnel: w464 -> [w474 w476]
              tunnel: [w474 w475] -> w463
              frame False {
              }
              frame True {
                n187 = call "Remove UI without races.vi"("error in"=w476, "user event ref"=w477, "sub panel ref in"=w478) -> ("error out"=w475:errorcluster)  [unwired: 7 in, 1 out]
              }
            }
            n188 = call <vilib>:"RemoveNode.vi"("error in"=w463, "node"=w468) -> ("error out"=w472:errorcluster, "node ID"=w473:string)  [unwired: 8 in]
            n189 = call <vilib>:"ClearTreeNode.vi"("error in"=w472, "tag"=w473, "tree reference"=w470) -> ("error out"=w471:errorcluster)  [unwired: 8 in]
          }
          frame True {
          }
        }
      }
      frame "PopulateTree" {
        n190 = Unbundle By Name(w491) -> ("current path"=w484:path, "root"=w488:T3)
        n191 = call <vilib>:"Summary.vi"("error in"=w486, "depth"=0 ("Depth"), "node self ref"=w488) -> ("error out"=w489:errorcluster, "summary"=w490:T19[])  [unwired: 7 in]
        n192 = Strip Path(path=w484) -> (name=w480:string)  [unwired: 1 out]
        n193 = call <vilib>:"RefreshEntireTree.vi"("calling VI in"=w481, "error in"=w489, "array"=w490, "tree ref in"=w485) -> ("error out"=w483:errorcluster)  [unwired: 7 in]
        n194 = property class="VI"(reference=w481, error in=w483, "Front Panel.Title"=w480) -> (error out=w482:errorcluster)  [unwired: 1 out]
      }
      frame "CleansubPanel" {
        n195 = Unbundle By Name(w495) -> ("user event ref"=w494:T4)
        n196 = call "Remove UI without races.vi"("error in"=w496, "user event ref"=w494, "sub panel ref in"=w492) -> ("error out"=w493:errorcluster)  [unwired: 7 in, 1 out]
      }
      frame "ActivateNode" {
        n197 = Unbundle By Name(w504) -> ("user event ref"=w501:T4)
        n198 = call <vilib>:"Set Busy.vi"("error in (no error)"=w507) -> ("error out"=w499:errorcluster)  [unwired: 9 in, 1 out]
        n199 = call <vilib>:"IDtoNode.vi"("error in"=w499, "ID"=w508) -> ("error out"=w500:errorcluster, "invalid Id"=w503:bool, "node ref"=w502:T3)  [unwired: 7 in]
        n200 = case shown="False" w503 {
          tunnel: w502 -> [w515 _]
          tunnel: [w516 w519] -> w498
          tunnel: w500 -> [w513 w520]
          tunnel: w505 -> [w511 _]
          tunnel: w501 -> [w512 w517]
          tunnel: w497 -> [w509 w518]
          frame False {
            n201 = call "Remove UI without races.vi"("error in"=w513, "user event ref"=w512, "sub panel ref in"=w509) -> ("error out"=w514:errorcluster, "sub panel ref out"=w510:refnum<vi>)  [unwired: 7 in]
            n202 = call <vilib>:"LoadNodeUI.vi"("user event out"=w512, "error in"=w514, "sub panel ref in"=w510, "main queue"=w511, "node"=w515) -> ("error out"=w516:errorcluster)  [unwired: 6 in]
          }
          frame True {
            n203 = call "Remove UI without races.vi"("error in"=w520, "user event ref"=w517, "sub panel ref in"=w518) -> ("error out"=w519:errorcluster)  [unwired: 7 in, 1 out]
          }
        }
        n204 = call <vilib>:"Unset Busy.vi"("error in (no error)"=w498) -> ("error out"=w506:errorcluster)  [unwired: 10 in]
      }
      frame "Move" {
        n205 = Unflatten From String(type=T11 {"node ref"=refnum, "new parent"=refnum} ("Cluster"), binary string=w531, error in (no error)=w530) -> (value=w526:T11, error out=w525:errorcluster)  [unwired: 2 in, 1 out]
        n206 = Unbundle By Name(w526) -> ("node ref"=w522:T3, "new parent"=w521:T3)
        n207 = call <vilib>:"MoveNode.vi"("error in"=w525, "new parent"=w521, "node"=w522) -> ("error out"=w523:errorcluster)  [unwired: 8 in]
        n208 = call <vilib>:"Send Local Message.vi"("message queue in"=w528, "message name"="PopulateTree", "error in"=w523) -> ("error out"=w529:errorcluster)  [unwired: 10 in, 2 out]
      }
      frame "RefreshNodeView" {
        # "This user event is used by editor nodes to update their subpanels when data in the tree changes."
        n209 = Unbundle By Name(w534) -> ("user event ref"=w533:T4)
        n210 = Generate User Event(user event=w533, event data cluster=T7 {"command"="Refresh", "data"=""} ("event data"), error in=w536) -> (error out=w535:errorcluster)  [unwired: 1 in, 1 out]
      }
    }
  }
  n211 = while "User Interface Event Handler" {
    tunnel: w12 -> [w542]
    tunnel: w10 -> [w538]
    stop <- w541 stop-if-true
    n212 = event shown="[1] \"View\": Shortcut Menu Selection (User)" {
      selector: _ -> [_ _ _ _ _ _ _ _ _]
      dyn-events: _ -> [_ _ _ _ _ _ _ _ _]
      timeout: _ -> [_ _ _ _ _ _ _ _ _]
      tunnel: w542 -> [w550 w576 w624 w664 w671 w698 w702 w712 w717]
      tunnel: [_ _ _ TRUE _ _ _ _ _] -> w541
      tunnel: [w550 w568 w626 w660 w671 w695 w702 w710 w716] -> w540
      tunnel: [w545 w569 w625 w661 w667 w694 w699 w708 w714] -> w539
      tunnel: w538 -> [w549 w574 w623 w662 w670 w693 w701 w709 w715]
      event "View": Shortcut Menu Activation? {
        n213 = event-data() -> ("CtlRef"=w556:refnum<vi>, "Coords"=w555:T20, "MenuRef"=w552:refnum<k9>)  [unwired: 1 in]
        n214 = invoke class="Tree (strict)" method="Point To Row Column"(reference=w556, error in=w549, "Point"=w555) -> (error out=w548:errorcluster, "Tag"=w554:string)  [unwired: 5 in, 6 out]
        n215 = call <vilib>:"IDtoNode.vi"("error in"=w548, "ID"=w554) -> ("error out"=w546:errorcluster, "invalid Id"=w551:bool, "node ref"=w553:T3)  [unwired: 7 in]
        n216 = case shown="False" w551 {
          selector: w551 -> [_ w566]
          tunnel: w553 -> [w560 _]
          tunnel: w552 -> [w559 _]
          tunnel: [w558 _] -> w547
          tunnel: [w557 _] -> w544
          tunnel: [_ w566] -> w543
          frame False {
            n217 = in-place {
              in-place-border: w559 -> [w563]
              in-place-border: [w561] -> w558
              n218 = in-place-dvr #7(w560) -> (w565:refnum<class "NISE_CEF_Node.lvclass">, w562:errorcluster)
              n219 = call-dynamic "ShortcutMenu.vi"("error in"=w562, "menu ref in"=w563, "node in"=w565) -> ("error out"=w561:errorcluster, "node out"=w564:refnum<class "NISE_CEF_Node.lvclass">)  [unwired: 6 in, 1 out]
              n220 = in-place-dvr #7(w564) -> (w557:errorcluster)  [unwired: 1 out]
            }
          }
          frame True {
          }
        }
        n221 = Merge Errors(w544, w547, w546) -> (w545:errorcluster)
        n222 = event-data("Discard?"=w543) -> ()  [unwired: 1 in, 1 out]
      }
      event "View": Shortcut Menu Selection (User) {
        # "=nodeID"
        n223 = event-data() -> ("ItemPath"=w572:string, "CtlRef"=w579:refnum<vi>, "Coords"=w580:T20)  [unwired: 1 in]
        n224 = invoke class="Tree (strict)" method="Point To Row Column"(reference=w579, error in=w574, "Point"=w580) -> (error out=w573:errorcluster, "Tag"=w575:string)  [unwired: 5 in, 6 out]
        n225 = Match Pattern(string=w572, regular expression=":") -> (before substring=w578:string, after substring=w577:string)  [unwired: 1 in, 2 out]
        n226 = case shown="Default" w578 {
          tunnel: w577 -> [_ _ _ w609 _]
          tunnel: w576 -> [w587 w598 w604 w611 w620]
          tunnel: w575 -> [w585 w592 w602 w610 w615]
          tunnel: [w584 w596 w601 w607 w618] -> w571
          tunnel: [w583 w595 w599 w605 w616] -> w570
          tunnel: w573 -> [w582 w591 w600 w606 w617]
          tunnel: w572 -> [_ w588 _ _ _]
          frame "Remove" {
            n227 = call <vilib>:"Send Local Message.vi"("message queue in"=w587, "message name"="RemoveNode" ("Message Name"), "message value"=w585, "error in"=w582) -> ("message queue out"=w584:T6, "error out"=w583:errorcluster)  [unwired: 9 in, 1 out]
          }
          frame Default {
            n228 = Bundle By Name(cluster=T9 {"node id"="", "RightClickPath"=""} ("input cluster"), "node id"=w592, "RightClickPath"=w588) -> (w593:T9)
            n229 = Flatten To String(anything=w593, error in (no error)=w591) -> (data string=w589:string, error out=w590:errorcluster)  [unwired: 2 in, 1 out]
            n230 = call <vilib>:"Send Local Message.vi"("message queue in"=w598, "message name"="HandleMenu" ("Message Name"), "message value"=w589, "error in"=w590) -> ("message queue out"=w596:T6, "error out"=w595:errorcluster)  [unwired: 9 in, 1 out]
          }
          frame "Duplicate" {
            n231 = call <vilib>:"Send Local Message.vi"("message queue in"=w604, "message name"="Duplicate" ("Message Name"), "message value"=w602, "error in"=w600) -> ("message queue out"=w601:T6, "error out"=w599:errorcluster)  [unwired: 9 in, 1 out]
          }
          frame "Add" {
            n232 = Bundle By Name(cluster=T10 {"node type"="", "to add to"=""} ("input cluster"), "node type"=w609, "to add to"=w610) -> (w612:T10)
            n233 = Flatten To String(anything=w612) -> (data string=w613:string)  [unwired: 3 in, 2 out]
            n234 = call <vilib>:"Send Local Message.vi"("message queue in"=w611, "message name"="AddNode" ("Message Name"), "message value"=w613, "error in"=w606) -> ("message queue out"=w607:T6, "error out"=w605:errorcluster)  [unwired: 9 in, 1 out]
          }
          frame "Async?" {
            n235 = call <vilib>:"Send Local Message.vi"("message queue in"=w620, "message name"="SetAsync" ("Message Name"), "message value"=w615, "error in"=w617) -> ("message queue out"=w618:T6, "error out"=w616:errorcluster)  [unwired: 9 in, 1 out]
          }
        }
        n236 = call <vilib>:"Send Local Message.vi"("message queue in"=w571, "message name"="RefreshNodeView", "error in"=w570) -> ("message queue out"=w568:T6, "error out"=w569:errorcluster)  [unwired: 10 in, 1 out]
      }
      event "View": Drop {
        n237 = event-data() -> ("CtlRef"=w622:refnum<vi>, "Coords"=w621:T20)  [unwired: 1 in]
        n238 = invoke class="Tree (strict)" method="Point To Row Column"(reference=w622, error in=w623, "Point"=w621) -> (reference out=w640:refnum<vi>, error out=w639:errorcluster, "Tag"=w636:string)  [unwired: 5 in, 5 out]
        n239 = call <vilib>:"ValidDragDrop.vi"("error in"=w639, "drag over"=w636, "tree ref in"=w640) -> ("error out"=w631:errorcluster, "accepted"=w634:bool, "drag"=w638:string, "tree ref out"=w641:refnum<vi>)  [unwired: 5 in]
        n240 = call <vilib>:"IDtoNode.vi"("error in"=w631, "ID"=w636) -> ("error out"=w632:errorcluster, "invalid Id"=w629:bool, "node ref"=w635:T3)  [unwired: 7 in]
        n241 = call <vilib>:"IDtoNode.vi"("error in"=w632, "ID"=w638) -> ("error out"=w630:errorcluster, "invalid Id"=w628:bool, "node ref"=w637:T3)  [unwired: 7 in]
        n242 = Compound Arithmetic op=AND(w634, invert w629, invert w628) -> (w633:bool)
        n243 = case shown="False" w633 {
          tunnel: w638 -> [_ w657]
          tunnel: w641 -> [_ w659]
          tunnel: [_ TRUE] -> w627
          tunnel: w636 -> [_ w655]
          tunnel: w624 -> [w643 w644]
          tunnel: [w643 w651] -> w626
          tunnel: [w642 w650] -> w625
          tunnel: w637 -> [_ w646]
          tunnel: w635 -> [_ w645]
          tunnel: w630 -> [w642 w647]
          frame False {
          }
          frame True {
            n244 = invoke class="Tree (strict)" method="Edit Tree Items.Move Item"(reference=w659, error in=w647, "tag"=w657, "New Parent"=w655) -> (error out=w648:errorcluster)  [unwired: 3 in, 6 out]
            n245 = Bundle By Name(cluster=T11 {"node ref"=refnum, "new parent"=refnum} ("Cluster"), "new parent"=w645, "node ref"=w646) -> (w654:T11)
            n246 = Flatten To String(anything=w654, error in (no error)=w648) -> (data string=w653:string, error out=w649:errorcluster)  [unwired: 2 in, 1 out]
            n247 = call <vilib>:"Send Local Message.vi"("message queue in"=w644, "message name"="Move", "message value"=w653, "error in"=w649) -> ("message queue out"=w651:T6, "error out"=w650:errorcluster)  [unwired: 9 in, 1 out]
          }
        }
        n248 = event-data("Accepted?"=w627) -> ()  [unwired: 1 in, 1 out]
      }
      event "Exit": Value Change {
        # "Exit the application                                           >> Stop this message generator loop    Cleaning errors if the other loop stop this one"
        n249 = event-data() -> ()  [unwired: 1 in, 1 out]
        n250 = call <vilib>:"Send Local Message.vi"("message queue in"=w664, "message name"="Close", "error in"=w662) -> ("message queue out"=w660:T6, "error out"=w665:errorcluster)  [unwired: 10 in, 1 out]
        n251 = call <vilib>:"Clear Errors.vi"("error in (no error)"=w665) -> ("error out"=w661:errorcluster)  [unwired: 6 in]
      }
      event "View": Drag Starting? {
        n252 = event-data() -> ("Data"=w677:T21, "CtlRef"=w679:refnum<vi>, "Coords"=w678:T20)  [unwired: 1 in]
        n253 = invoke class="Tree (strict)" method="Point To Row Column"(reference=w679, error in=w670, "Point"=w678) -> (error out=w669:errorcluster, "Tag"=w676:string)  [unwired: 5 in, 6 out]
        n254 = call <vilib>:"IDtoNode.vi"("error in"=w669, "ID"=w676) -> ("error out"=w668:errorcluster, "invalid Id"=w675:bool, "node ref"=w674:T3)  [unwired: 7 in]
        n255 = case shown="False" w675 {
          tunnel: w674 -> [w685 _]
          tunnel: [w682 TRUE ("Removable")] -> w672
          tunnel: w668 -> [w681 w691]
          tunnel: [w680 w691] -> w667
          frame False {
            n256 = in-place {
              in-place-border: [w688] -> w684
              in-place-border: w681 -> [w687]
              in-place-border: [w686] -> w680
              n257 = in-place-dvr #8(w685) -> (w690:refnum<class "NISE_CEF_Node.lvclass">)  [unwired: 1 out]
              n258 = call-dynamic "EditOptions.vi"("error in"=w687, "node in"=w690) -> ("error out"=w686:errorcluster, "edit options"=w688:T22, "node out"=w689:refnum<class "NISE_CEF_Node.lvclass">)  [unwired: 6 in, 1 out]
              n259 = in-place-dvr #8(w689) -> ()  [unwired: 2 out]
            }
            n260 = Unbundle By Name(w684) -> ("movable"=w683:bool)
            n261 = Not(x=w683) -> (.not. x?=w682:bool)
          }
          frame True {
          }
        }
        n262 = event-data("Data"=w677, "Drag Mode"=enum32{"copy or move", "copy only", "move only"}."move only", "Discard?"=w672) -> ()  [unwired: 1 in, 1 out]
      }
      event "View": Value Change {
        n263 = event-data() -> ("NewVal"=w696:string)  [unwired: 1 in]
        n264 = call <vilib>:"Send Local Message.vi"("message queue in"=w698, "message name"="ActivateNode" ("Message Name"), "message value"=w696, "error in"=w693) -> ("message queue out"=w695:T6, "error out"=w694:errorcluster)  [unwired: 9 in, 1 out]
      }
      event "View": event type 3.0.xa000003a {
        n265 = event-data() -> ("CtlRef"=w707:refnum<vi>, "Coords"=w704:T20)  [unwired: 1 in]
        n266 = invoke class="Tree (strict)" method="Point To Row Column"(reference=w707, error in=w701, "Point"=w704) -> (reference out=w706:refnum<vi>, error out=w700:errorcluster, "Tag"=w705:string)  [unwired: 5 in, 5 out]
        n267 = call <vilib>:"ValidDragDrop.vi"("error in"=w700, "drag over"=w705, "tree ref in"=w706) -> ("error out"=w699:errorcluster, "accepted"=w703:bool)  [unwired: 5 in, 2 out]
        n268 = event-data("Accepted?"=w703) -> ()  [unwired: 1 in, 1 out]
      }
      event Panel Close? {
        # "Intercepts the upper right close panel operation to allow a smooth shutdown as opposed to immediately killing the app."
        n269 = event-data() -> ()  [unwired: 1 in, 1 out]
        n270 = call <vilib>:"Send Local Message.vi"("message queue in"=w712, "message name"="Close?", "error in"=w709) -> ("message queue out"=w710:T6, "error out"=w708:errorcluster)  [unwired: 10 in, 1 out]
        n271 = event-data("Discard?"=TRUE) -> ()  [unwired: 1 in, 1 out]
      }
      event Menu Selection (User) {
        n272 = event-data() -> ("ItemPath"=w718:string)  [unwired: 1 in]
        n273 = case shown="\"_File:Save As...\"" w718 {
          tunnel: w717 -> [w720 w726 w731 w736 w741 w746 w755 w760 w766 w770]
          tunnel: [w720 w722 w727 w732 w737 w742 w752 w757 w763 w769] -> w716
          tunnel: w715 -> [w719 w724 w729 w734 w739 w744 w751 w758 w764 w768]
          tunnel: [w719 w723 w728 w733 w738 w743 w749 w756 w762 w767] -> w714
          frame Default {
            n274 = One Button Dialog(message="Unknown Menu Option") -> ()  [unwired: 1 in, 1 out]
          }
          frame "_File:_New" {
            n275 = call <vilib>:"Send Local Message.vi"("message queue in"=w726, "message name"="New?" ("Message Name"), "error in"=w724) -> ("message queue out"=w722:T6, "error out"=w723:errorcluster)  [unwired: 10 in, 1 out]
          }
          frame "_File:_Open" {
            n276 = call <vilib>:"Send Local Message.vi"("message queue in"=w731, "message name"="Open?" ("Message Name"), "error in"=w729) -> ("message queue out"=w727:T6, "error out"=w728:errorcluster)  [unwired: 10 in, 1 out]
          }
          frame "_File:_Save" {
            n277 = call <vilib>:"Send Local Message.vi"("message queue in"=w736, "message name"="Save" ("Message Name"), "error in"=w734) -> ("message queue out"=w732:T6, "error out"=w733:errorcluster)  [unwired: 10 in, 1 out]
          }
          frame "_File:Save As..." {
            n278 = call <vilib>:"Send Local Message.vi"("message queue in"=w741, "message name"="SaveAs" ("Message Name"), "error in"=w739) -> ("message queue out"=w737:T6, "error out"=w738:errorcluster)  [unwired: 10 in, 1 out]
          }
          frame "_File:_Exit" {
            n279 = call <vilib>:"Send Local Message.vi"("message queue in"=w746, "message name"="Close?" ("Message Name"), "error in"=w744) -> ("message queue out"=w742:T6, "error out"=w743:errorcluster)  [unwired: 10 in, 1 out]
          }
          frame "_Tools:Multiple Parameter Editor" {
            n280 = call <vilib>:"Send Local Message.vi"("message queue in"=w755, "message name"="CleansubPanel", "error in"=w751) -> ("message queue out"=w754:T6, "error out"=w750:errorcluster)  [unwired: 10 in, 1 out]
            n281 = call <vilib>:"Send Local Message.vi"("message queue in"=w754, "message name"="Custom View", "message value"="Multiple Parameter Editor" ("Message Name"), "error in"=w750) -> ("message queue out"=w752:T6, "error out"=w749:errorcluster)  [unwired: 9 in, 1 out]
          }
          frame "_Tools:Test" {
            n282 = call <vilib>:"Send Local Message.vi"("message queue in"=w760, "message name"="Test", "error in"=w758) -> ("message queue out"=w757:T6, "error out"=w756:errorcluster)  [unwired: 10 in, 1 out]
          }
          frame "_Tools:Refresh Plugins" {
            n283 = call <vilib>:"Send Local Message.vi"("message queue in"=w766, "message name"="FindPluginNodes", "message value"="Refresh", "error in"=w764) -> ("message queue out"=w763:T6, "error out"=w762:errorcluster)  [unwired: 9 in, 1 out]
          }
          frame "_Tools:Edit Plugin Search Paths" {
            n284 = call <vilib>:"Send Local Message.vi"("message queue in"=w770, "message name"="Edit Plugin Search Paths", "error in"=w768) -> ("message queue out"=w769:T6, "error out"=w767:errorcluster)  [unwired: 10 in, 1 out]
          }
        }
      }
    }
    n285 = call "send error message.vi"("error in"=w539, "message queue in"=w540) -> ()  [unwired: 9 in, 1 out]
  }
